vi "Execute Turn.vi"(8 "error in":errorcluster, 11 "Reversi in":refnum<class "Reversi.lvclass">) -> (0 "error out":errorcluster, 3 "Reversi out":refnum<class "Reversi.lvclass">)   [LabVIEW 2020, in "Reversi.lvlib" / "Reversi.lvclass"]
uses:
  Reversi.lvclass
  Reversi.lvclass/Reversi.ctl
  Space Cluster.ctl
  Space Coordinates.ctl
  Space Ring.ctl
  Player/Player.lvclass
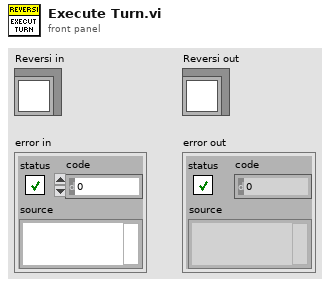
[diagram p1: front panel]
types:
  T1 = typedef "Reversi.lvlib/Reversi.lvclass/Space Ring.ctl" = u16
  T2 = typedef "Reversi.lvlib/Reversi.lvclass/Turn Enum.ctl" = enum16{"Black", "White"}
  T3 = typedef "Reversi.lvlib/Reversi.lvclass/Space Cluster.ctl" = cluster{"Coordinates":T4, "Ring":T1}
  T4 = typedef "Reversi.lvlib/Reversi.lvclass/Space Coordinates.ctl" = cluster{"Row":i32, "Column":i32}
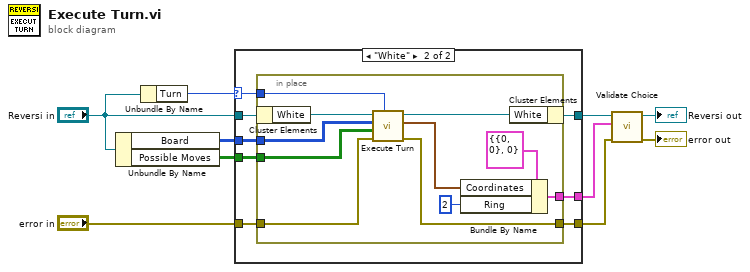
[diagram p0: block diagram]
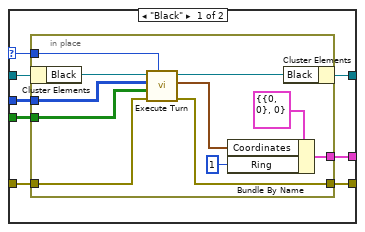
[diagram p2: hidden frame]
diagram:
  n1 = Unbundle By Name("Reversi in") -> ("Board"=w7:T1[][], "Possible Moves"=w6:bool[][])
  n2 = Unbundle By Name("Reversi in") -> ("Turn"=w1:T2)
  n3 = case shown="\"White\"" w1 {
    selector: w1 -> [w11 w30]
    tunnel: "Reversi in" -> [w16 w35]
    tunnel: w7 -> [w15 w34]
    tunnel: w6 -> [w14 w33]
    tunnel: "error in" -> [w18 w37]
    tunnel: [w13 w32] -> w5
    tunnel: [w12 w31] -> w4
    tunnel: [w17 w36] -> w9
    frame "Black" {
      n4 = in-place {
        in-place-border: w15 -> [w25]
        in-place-border: w14 -> [w24]
        in-place-border: w18 -> [w29]
        in-place-border: [w28] -> w17
        in-place-border: [w20] -> w12
        in-place-border: w11 -> [w19]
        n5 = in-place-cluster #1(w16) -> ("Black"=w27:refnum<class "Player.lvclass">)
        n6 = call-dynamic "Execute Turn.vi"("Player Color"=w19, "error in"=w29, "Possible Moves"=w24, "Board"=w25, "Player in"=w27) -> ("error out"=w28:errorcluster, "Choice Coordinates"=w22:T4, "Player out"=w26:refnum<class "Player.lvclass">)  [unwired: 4 in]
        n7 = Bundle By Name(cluster=T3 {"Coordinates"={"Row"=0, "Column"=0}, "Ring"=0} ("Space"), "Coordinates"=w22, "Ring"=T1 1) -> (w20:T3)
        n8 = in-place-cluster #1("Black"=w26) -> (w13:refnum<class "Reversi.lvclass">)
      }
    }
    frame "White" {
      n9 = in-place {
        in-place-border: w34 -> [w44]
        in-place-border: w33 -> [w40]
        in-place-border: w37 -> [w48]
        in-place-border: [w47] -> w36
        in-place-border: [w41] -> w31
        in-place-border: w30 -> [w38]
        n10 = in-place-cluster #2(w35) -> ("White"=w46:refnum<class "Player.lvclass">)
        n11 = call-dynamic "Execute Turn.vi"("Player Color"=w38, "error in"=w48, "Possible Moves"=w40, "Board"=w44, "Player in"=w46) -> ("error out"=w47:errorcluster, "Choice Coordinates"=w39:T4, "Player out"=w45:refnum<class "Player.lvclass">)  [unwired: 4 in]
        n12 = Bundle By Name(cluster=T3 {"Coordinates"={"Row"=0, "Column"=0}, "Ring"=0} ("Space"), "Coordinates"=w39, "Ring"=T1 2) -> (w41:T3)
        n13 = in-place-cluster #2("White"=w45) -> (w32:refnum<class "Reversi.lvclass">)
      }
    }
  }
  n14 = call "Validate Choice.vi"("error in (no error)"=w9, "Choice"=w4, "Reversi in"=w5) -> ("error out"=→"error out":errorcluster, "Reversi out"=→"Reversi out":refnum<class "Reversi.lvclass">)  [unwired: 7 in]
